vi "报警设置.vi"() -> ()   [LabVIEW 2016, in "环境动力监测库.lvlib"]
uses:
  <vilib>/Utility/config.llb/NI_LVConfig.lvlib
panel:
  out "MPPT24低压报警阈值 V":dbl=11.0
  out "MPPT12低压报警阈值 V":dbl=11.0
  in  "布尔":bool
  # "参数设置"
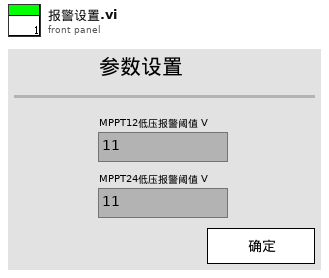
[diagram p1: front panel]
types:
  T1 = typedef "NI_LVConfig.lvlib/Config Data RefNum.ctl" = refnum<k1>
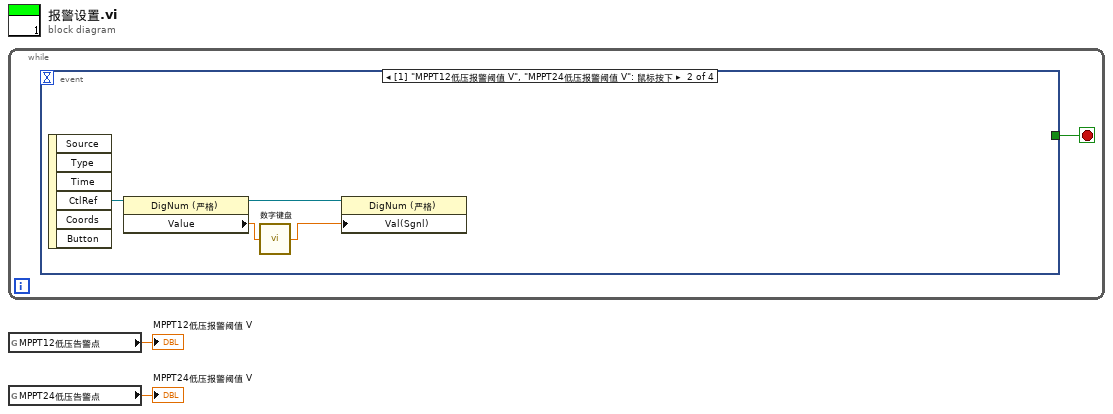
[diagram p0: block diagram]
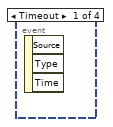
[diagram p2: hidden frame]
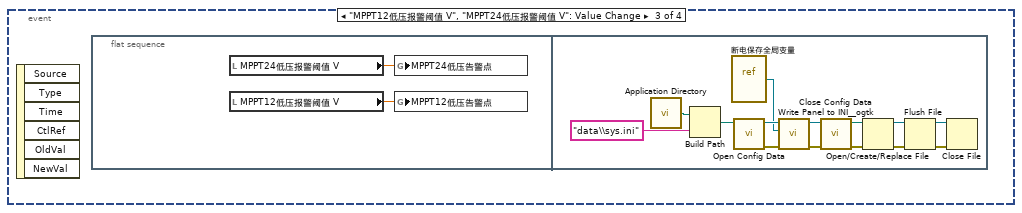
[diagram p3: hidden frame]
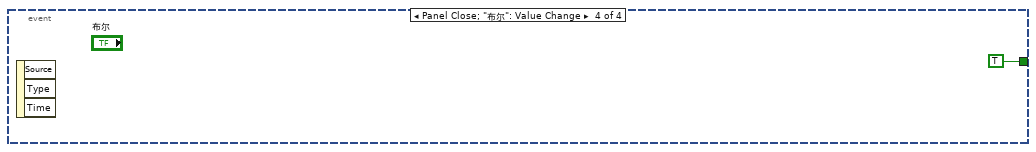
[diagram p4: hidden frame]
diagram:
  n1 = while {
    stop <- w3 stop-if-true
    n2 = event shown="[1] \"MPPT12低压报警阈值 V\", \"MPPT24低压报警阈值 V\": 鼠标按下" {
      selector: _ -> [_ _ _ _]
      dyn-events: _ -> [_ _ _ _]
      timeout: _ -> [_ _ _ _]
      tunnel: [_ _ _ TRUE] -> w3
      event Timeout {
        n3 = event-data() -> ()  [unwired: 1 in, 3 out]
      }
      event "MPPT12低压报警阈值 V", "MPPT24低压报警阈值 V": Mouse Down {
        n4 = event-data() -> ("CtlRef"=w6:refnum<vi>)  [unwired: 1 in, 5 out]
        n5 = property class="DigNum (严格)"(reference=w6) -> (reference out=w7:refnum<vi>, "Value"=w5:dbl)  [unwired: 1 in, 1 out]
        n6 = call "数字键盘.vi"("OldNumber"=w5) -> ("NewNumber"=w4:sgl)
        n7 = property class="DigNum (严格)"(reference=w7, "Val(Sgnl)"=w4) -> ()  [unwired: 1 in, 2 out]
      }
      event "MPPT12低压报警阈值 V", "MPPT24低压报警阈值 V": Value Change {
        n8 = event-data() -> ()  [unwired: 1 in, 6 out]
        n9 = flat-sequence {
          frame #0 {
            n10 = local read "MPPT24低压报警阈值 V"() -> (w8:dbl)
            n11 = local read "MPPT12低压报警阈值 V"() -> (w9:dbl)
            n12 = global write "断电保存全局变量.vi" "MPPT24低压告警点"(w8) -> ()
            n13 = global write "断电保存全局变量.vi" "MPPT12低压告警点"(w9) -> ()
          }
          frame #1 {
            n14 = call <vilib>:"Application Directory.vi"() -> ("Application Directory"=w23:path)
            n15 = Build Path(base path=w23, name or relative path="data\\sys.ini" ("名称或相对路径")) -> (appended path=w21:path)
            n16 = vi-ref "断电保存全局变量.vi"() -> (w19:refnum<vi>)
            n17 = call <vilib>:"Open Config Data.vi"("configuration file path"=w21) -> ("error out"=w17:errorcluster, "refnum"=w20:T1)  [unwired: 8 in, 1 out]
            n18 = call <userlib>:"Write Panel to INI__ogtk.vi"("error in (no error)"=w17, "VI ref"=w19, "refnum"=w20) -> ("error out"=w16:errorcluster, "refnum out"=w18:T1)  [unwired: 7 in]
            n19 = call <vilib>:"Close Config Data.vi"("error in (no error)"=w16, "refnum"=w18) -> ("error out"=w11:errorcluster, "file path"=w10:path)  [unwired: 8 in]
            n20 = Open/Create/Replace File(file path (use dialog)=w10, error in=w11) -> (refnum out=w14:refnum<file>, error out=w15:errorcluster)  [unwired: 4 in, 1 out]
            n21 = Flush File(refnum=w14, error in=w15) -> (refnum out=w13:refnum<file>, error out=w12:errorcluster)
            n22 = Close File(refnum=w13, error in=w12) -> ()  [unwired: 2 out]
          }
        }
      }
      event Panel Close; "布尔": Value Change {
        n23 = event-data() -> ()  [unwired: 1 in, 3 out]
      }
    }
  }
  n24 = global read "断电保存全局变量.vi" "MPPT12低压告警点"() -> (→"MPPT12低压报警阈值 V":dbl)
  n25 = global read "断电保存全局变量.vi" "MPPT24低压告警点"() -> (→"MPPT24低压报警阈值 V":dbl)
